vi "Initialize.vi"(7 "Serial Configuration":T1={"Baud Rate"=9600, "Parity"=0, "Data Bits"=8, "Stop Bits"=10, "Flow Control"=0} {"Flow Control" items=["None", "XON/XOFF", "RTS/CTS", "XON/XOFF & RTS/CTS", "DTR/DSR", "XON/XOFF & DTR/DSR"]; "Stop Bits" items=["1.0"=10, "1.5"=15, "2.0"=20]; "Data Bits" items=["7"=7, "8"=8]; "Parity" items=["None", "Odd", "Even", "Mark", "Space"]; "Baud Rate" items=["300"=300, "600"=600, "1200"=1200, "2400"=2400, "4800"=4800, "9600"=9600, "19200"=19200]}, 8 "error in":errorcluster, 9 "Reset":bool, 10 "ID Query":bool, 11 "VISA resource name":refnum<visa-resource-name>) -> (0 "error out":errorcluster, 3 "VISA resource name out":refnum<visa-resource-name>)   [LabVIEW 2015, in "IT6700H.lvlib"]
doc: "Establishes communication with the instrument and optionally performs an instrument identification query and/or an instrument reset. It also places the instrument in a default state needed for other instrument driver operations. Therefore, call this VI before calling other instrument driver VIs for this instrument. Generally, you need to call the <b>Initialize</b> VI only once at the beginning of an application."
uses:
  <instrlib>/IT6700H/IT6700H.lvlib
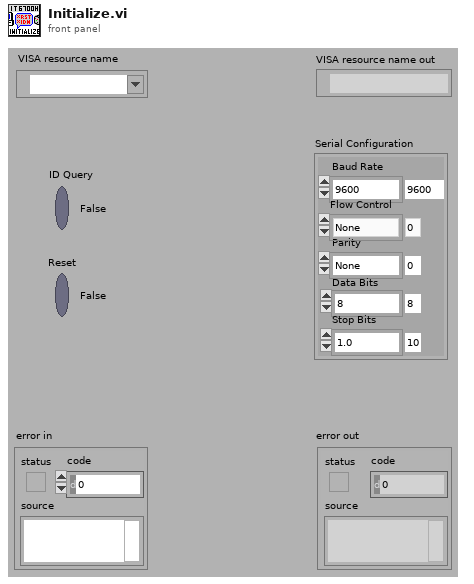
[diagram p1: front panel]
types:
  T1 = cluster{"Baud Rate":u32, "Parity":u16, "Data Bits":u16, "Stop Bits":u16, "Flow Control":u16}
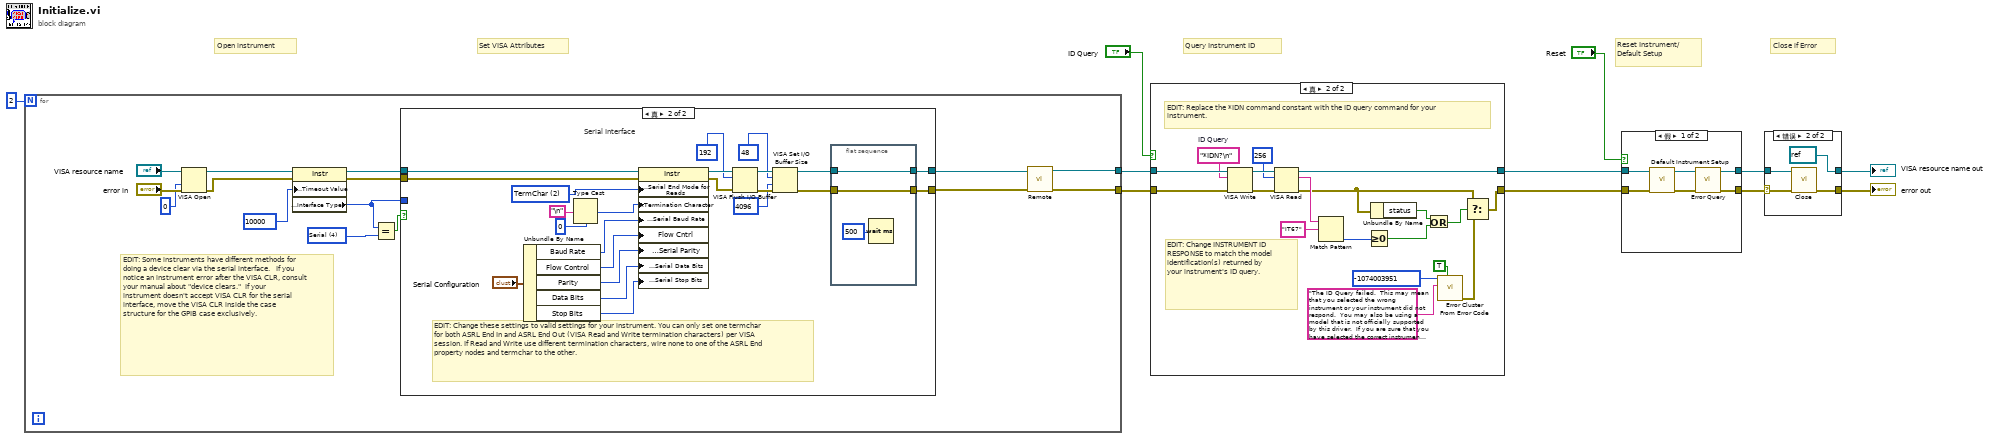
[diagram p0: block diagram]
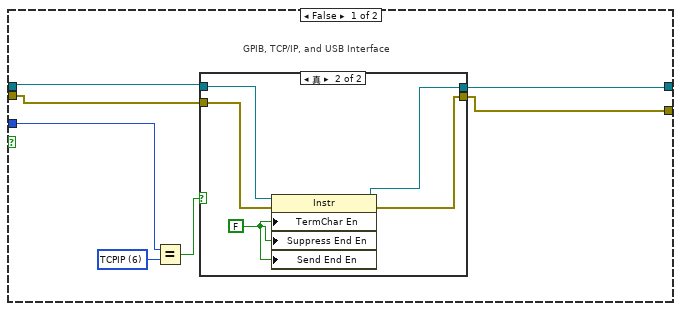
[diagram p2: hidden frame]
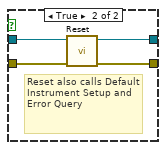
[diagram p5: hidden frame]
diagram:
  # "Set VISA Attributes"
  # "Close if Error"
  # "Query Instrument ID"
  # "Reset Instrument/\nDefault Setup"
  # "Open instrument"
  n1 = for {
    N: 2 -> [_]
    tunnel: [w13] -> w9
    tunnel: [w12] -> w8
    w20 = u16 4 items=["GPIB"=1, "VXI"=2, "GPIB-VXI"=3, "Serial"=4, "PXI"=5, "TCPIP"=6, "USB"=7] ("Interface Information:Interface Type")
    # "EDIT: Some instruments have different methods for doing a device clear via the serial interface.   If you notice an instrument error after the VISA CLR, consult your manual about \"device clears.\"  If your instrument doesn't accept VISA CLR for the serial interface, move the VISA CLR inside the case  structure for the GPIB case exclusively."
    n2 = VISA Open(access mode=u32 0, error in (no error)="error in", VISA resource name="VISA resource name") -> (VISA resource name=w18:refnum<visa-resource-name>, error out=w17:errorcluster)  [unwired: 2 in]
    n3 = property class="Instr"(reference=w18, error in=w17, "General Settings:Timeout Value"=u32 10000) -> (reference out=w23:refnum<visa-resource-name>, error out=w22:errorcluster, "Interface Information:Interface Type"=w16:u16)
    n4 = Equal?(x=w16, y=w20) -> (x = y?=w21:bool)
    n5 = case shown="真" w21 {
      tunnel: [w28 w44] -> w15
      tunnel: [w27 w42] -> w14
      tunnel: w23 -> [w31 w48]
      tunnel: w22 -> [w30 w47]
      tunnel: w16 -> [w29 _]
      frame False {
        w33 = u16 6 items=["GPIB"=1, "VXI"=2, "GPIB-VXI"=3, "Serial"=4, "PXI"=5, "TCPIP"=6, "USB"=7] ("Interface Information:Interface Type")
        # "GPIB, TCP/IP, and USB Interface"
        n6 = Equal?(x=w29, y=w33) -> (x = y?=w32:bool)
        n7 = case shown="真" w32 {
          tunnel: [w35 w40] -> w28
          tunnel: [w34 w39] -> w27
          tunnel: w31 -> [w35 w38]
          tunnel: w30 -> [w34 w37]
          frame False {
          }
          frame True {
            w36 = FALSE
            n8 = property class="Instr"(reference=w38, error in=w37, "TermChar En"=w36, "Suppress End En"=w36, "Send End En"=w36) -> (reference out=w40:refnum<visa-resource-name>, error out=w39:errorcluster)
          }
        }
      }
      frame True {
        w41 = u16 2 items=["None", "LastBit", "TermChar"] ("Serial Settings:Serial End Mode for Reads")
        # "EDIT: Change these settings to valid settings for your instrument. You can only set one termchar for both ASRL End In and ASRL End Out (VISA Read and Write termination characters) per VISA session. If Read and Write use different termination characters, wire none to one of the ASRL End property nodes and termchar to the other."
        # "Serial Interface"
        n9 = Unbundle By Name("Serial Configuration") -> ("Baud Rate"=w53:u32, "Flow Control"=w46:u16, "Parity"=w51:u16, "Data Bits"=w52:u16, "Stop Bits"=w49:u16)
        n10 = Type Cast(type=u8 0, x="\n" ("Line Feed Constant")) -> (*(type *) &x=w54:u8)
        n11 = property class="Instr"(reference=w48, error in=w47, "Serial Settings:Serial End Mode for Reads"=w41, "Message Based Settings:Termination Character"=w54, "Serial Settings:Serial Baud Rate"=w53, "Flow Cntrl"=w46, "Serial Settings:Serial Parity"=w51, "Serial Settings:Serial Data Bits"=w52, "Serial Settings:Serial Stop Bits"=w49) -> (reference out=w60:refnum<visa-resource-name>, error out=w62:errorcluster)
        n12 = VISA Flush I/O Buffer(VISA resource name=w60, mask (16)=u16 192, error in (no error)=w62) -> (VISA resource name out=w63:refnum<visa-resource-name>, error out=w61:errorcluster)
        n13 = VISA Set I/O Buffer Size(VISA resource name=w63, mask (16)=u16 48, size (4096)=u32 4096 ("size (0)"), error in (no error)=w61) -> (VISA resource name out=w45:refnum<visa-resource-name>, error out=w43:errorcluster)
        n14 = flat-sequence {
          tunnel: w45 -> [w66]
          tunnel: [w66] -> w44
          tunnel: w43 -> [w65]
          tunnel: [w65] -> w42
          frame #0 {
            n15 = Wait (ms)(milliseconds to wait=500) -> ()  [unwired: 1 out]
          }
        }
      }
    }
    n16 = call <instrlib>:"Remote.vi"("error in"=w14, "VISA resource name"=w15) -> ("error out"=w12:errorcluster, "VISA resource name out"=w13:refnum<visa-resource-name>)  [unwired: 8 in]
  }
  n17 = case shown="真" "ID Query" {
    tunnel: [w67 w87] -> w3
    tunnel: [w68 w84] -> w2
    tunnel: w9 -> [w68 w85]
    tunnel: w8 -> [w67 w86]
    frame False {
    }
    frame True {
      w78 = "*IDN?\n"  # ID Query
      # "EDIT: Replace the *IDN command constant with the ID query command for your instrument."
      # "EDIT: Change INSTRUMENT ID RESPONSE to match the model identification(s) returned by your instrument's ID query."
      n18 = VISA Write(VISA resource name=w85, write buffer=w78, error in (no error)=w86) -> (VISA resource name out=w82:refnum<visa-resource-name>, error out=w81:errorcluster)  [unwired: 1 out]
      n19 = VISA Read(VISA resource name=w82, byte count=u32 256, error in (no error)=w81) -> (VISA resource name out=w84:refnum<visa-resource-name>, read buffer=w83:string, error out=w72:errorcluster)  [unwired: 1 out]
      n20 = Match Pattern(string=w83, regular expression="IT67") -> (offset past match=w73:i32)  [unwired: 1 in, 3 out]
      n21 = Greater Or Equal To 0?(x=w73) -> (x >= 0?=w70:bool)
      n22 = Unbundle By Name(w72) -> ("status"=w71:bool)
      n23 = Or(x=w71, y=w70) -> (x .or. y?=w69:bool)
      n24 = call <vilib>:"Error Cluster From Error Code.vi"("show call chain? (False)"=TRUE, "error message (\"\")"="The ID Query failed.  This may mean that you selected the wrong instrument or your instrument did not respond.  You may also be using a model that is not officially supported by this driver.  If you are sure that you have selected the correct instrument and it is responding, try disabling the ID Query." ("Source (VI Name)"), "error code (0)"=-1074003951 ("Code")) -> ("error out"=w77:errorcluster)  [unwired: 6 in]
      n25 = Select(t=w72, s=w69, f=w77) -> (s? t:f=w87:errorcluster)
    }
  }
  n26 = case shown="假" "Reset" {
    tunnel: w3 -> [w88 w94]
    tunnel: [w92 w97] -> w4
    tunnel: w2 -> [w89 w95]
    tunnel: [w93 w96] -> w5
    frame False {
      n27 = call <instrlib>:"Default Instrument Setup.vi"("error in"=w88, "VISA resource name"=w89) -> ("error out"=w91:errorcluster, "VISA resource name out"=w90:refnum<visa-resource-name>)  [unwired: 8 in]
      n28 = call <instrlib>:"Error Query.vi"("error in"=w91, "VISA resource name"=w90) -> ("error out"=w92:errorcluster, "VISA resource name out"=w93:refnum<visa-resource-name>)  [unwired: 6 in, 2 out]
    }
    frame True {
      # "Reset also calls Default Instrument Setup and Error Query"
      n29 = call <instrlib>:"Reset.vi"("error in"=w94, "VISA resource name"=w95) -> ("error out"=w97:errorcluster, "VISA resource name out"=w96:refnum<visa-resource-name>)  [unwired: 8 in]
    }
  }
  n30 = case shown="错误" w4 {
    selector: w4 -> [w98 w101]
    tunnel: w5 -> [w99 w102]
    tunnel: [w99 refnum<visa-resource-name> refnum ("VISA resource name out")] -> w7
    tunnel: [w98 w103] -> w6
    frame No Error {
    }
    frame Error {
      n31 = call <instrlib>:"Close.vi"("error in"=w101, "VISA resource name"=w102) -> ("error out"=w103:errorcluster)  [unwired: 9 in]
    }
  }
  "VISA resource name out" <- w7
  "error out" <- w6
